vi "UI Event Handler.vi"() -> ()   [LabVIEW 2012]
uses:
  <vilib>/Utility/miscctls.llb/LVPoint32TypeDef.ctl
panel:
  out "当前时间":timestamp
  in  "时间检查":bool
  out "坐标":T1
  out "迭代":i32
  in  "停止":bool
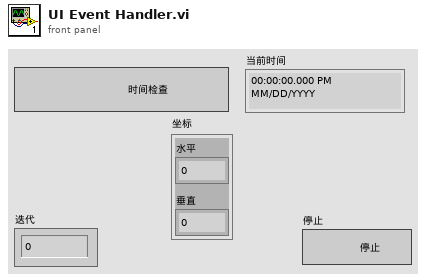
[diagram p1: front panel]
types:
  T1 = typedef "LVPoint32TypeDef.ctl" = cluster{"Horizontal":i32, "Vertical":i32}
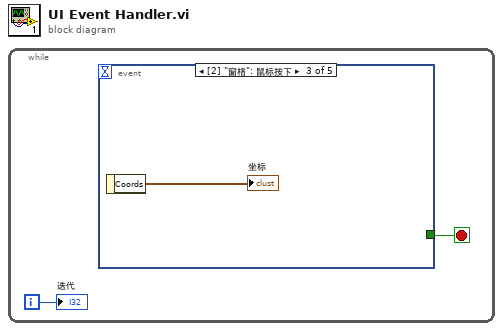
[diagram p0: block diagram]
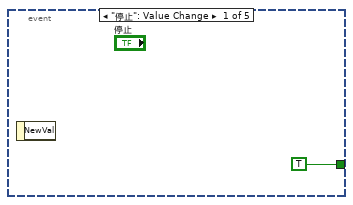
[diagram p2: hidden frame]
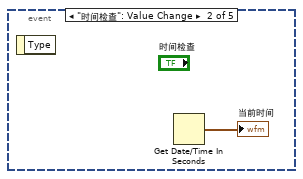
[diagram p3: hidden frame]
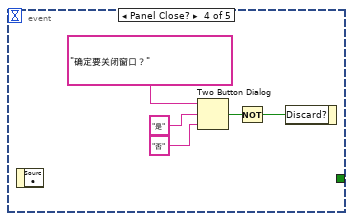
[diagram p4: hidden frame]
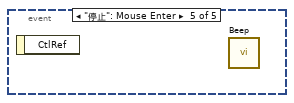
[diagram p5: hidden frame]
diagram:
  n1 = while {
    i -> [w2]
    stop <- w1 stop-if-true
    n2 = event shown="[2] \"窗格\": 鼠标按下" {
      selector: _ -> [_ _ _ _ _]
      dyn-events: _ -> [_ _ _ _ _]
      timeout: _ -> [_ _ _ _ _]
      tunnel: [TRUE _ _ _ _] -> w1
      event "停止": Value Change {
        n3 = event-data ("事件数据节点")() -> ()  [unwired: 1 in, 1 out]
      }
      event "时间检查": Value Change {
        n4 = event-data ("事件数据节点")() -> ()  [unwired: 1 in, 1 out]
        n5 = Get Date/Time In Seconds ("获取日期/时间（秒）")() -> (seconds since 1Jan1904=→"当前时间":timestamp)
      }
      event Mouse Down {
        n6 = event-data ("事件数据节点")() -> ("Coords"=→"坐标":T1)  [unwired: 1 in]
      }
      event Panel Close? {
        n7 = event-data ("事件数据节点")() -> ()  [unwired: 1 in, 1 out]
        n8 = Two Button Dialog ("双按钮对话框")(message="确定要关闭窗口？" ("消息"), 1:"否" ("T按钮名称（“确定”）"), 2:"是" ("F按钮名称（“取消”）")) -> (T button?=w10:bool)
        n9 = Not ("非")(x=w10) -> (.not. x?=w6:bool)
        n10 = event-data ("事件过滤节点")("Discard?"=w6) -> ()  [unwired: 1 in, 1 out]
      }
      event "停止": Mouse Enter {
        n11 = event-data ("事件数据节点")() -> ()  [unwired: 1 in, 1 out]
        n12 = call <vilib>:"Beep.vi"() -> ()  [unwired: 12 in]
      }
    }
    "迭代" <- w2
  }
